vi "Test - Draw Filled Triangle.vi"() -> ()   [LabVIEW 2020, in "Raster.lvlib"]
uses:
  Raster.lvlib
  Point 2D.ctl
  Screen Dimensions.ctl
  <vilib>/Utility/High Resolution Relative Seconds.vi
  Utility/Utility.lvlib
panel:
  in  "Point 3":T1={"x"=0, "y"=200}
  in  "Point 2":T1={"x"=100, "y"=100}
  in  "Point 1":T1
  out "Time [s]":dbl format="%.3p"
  out "new picture":picture
  # "(0,0)"
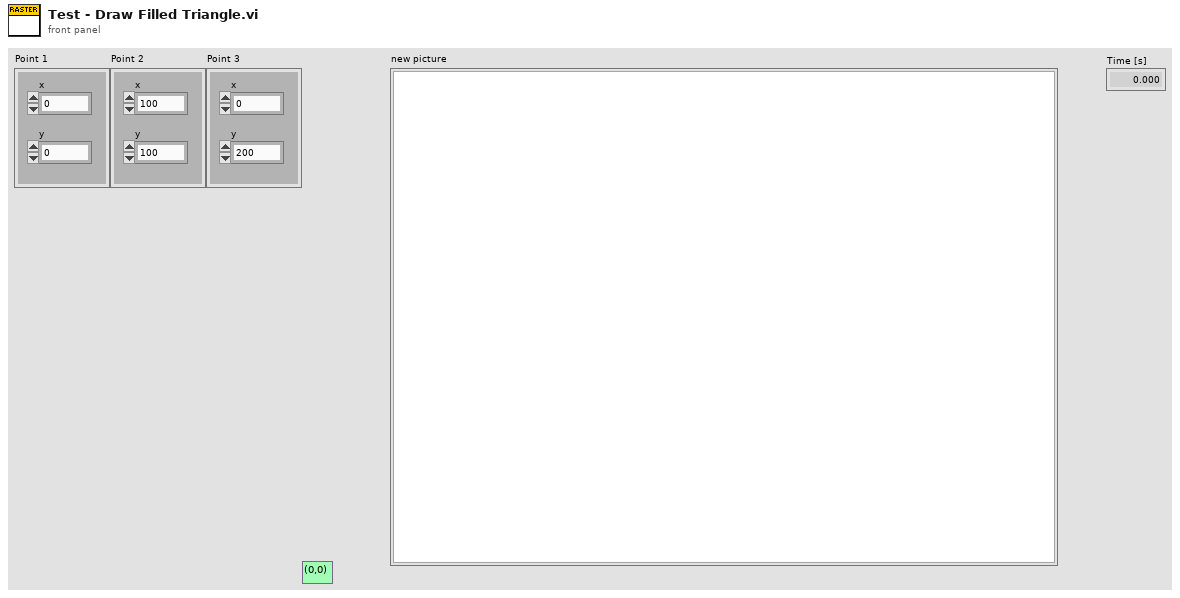
[diagram p1: front panel]
types:
  T1 = typedef "Raster.lvlib/Point 2D.ctl" = cluster{"x":i32, "y":i32}
  T2 = typedef "Raster.lvlib/Screen Dimensions.ctl" = cluster{"Width":u32, "Height":u32}
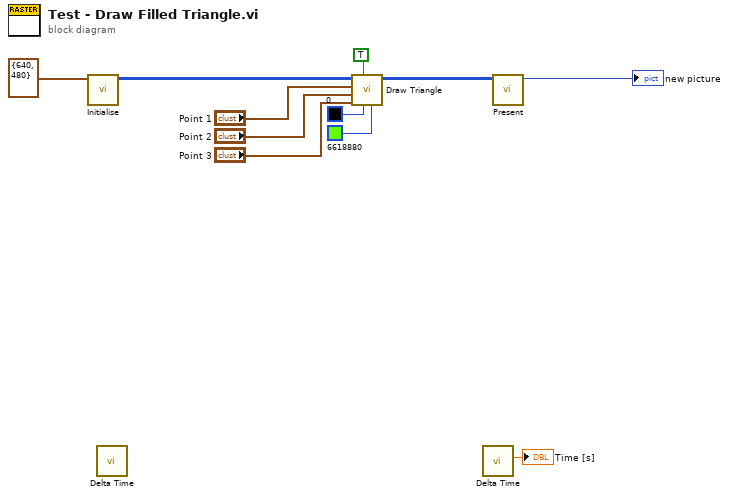
[diagram p0: block diagram]
diagram:
  n1 = call "Initialise.vi"("Screen Dimensions"=T2 {"Width"=640, "Height"=480}) -> ("Pixel Data out"=w6:u32[][])  [unwired: 10 in]
  n2 = call "Delta Time.vi"() -> ()  [unwired: 10 in, 2 out]
  n3 = call "Draw Triangle.vi"("Fill Colour"=u32 6618880, "Line Colour"=u32 0, "Fill (F)"=TRUE, "Point 3"="Point 3", "Point 2"="Point 2", "Point 1"="Point 1", "Pixel Data in"=w6) -> ("Pixel Data out"=w5:u32[][])  [unwired: 4 in]
  n4 = call "Delta Time.vi"() -> ("Delta Time [s]"=→"Time [s]":dbl)  [unwired: 10 in, 1 out]
  n5 = call "Present.vi"("Pixel Data in"=w5) -> ("2D Picture"=→"new picture":picture)  [unwired: 10 in]
